vi "FC_Parse_Comp_Info.vi"(8 "Error In":errorcluster, 10 "All Competition Data":string) -> (0 "Error Out":errorcluster, 2 "Comp Data Cluster":T1)   [LabVIEW 2014, in "FC_FIRST Client.lvlib"]
doc: "This VI parses the data of a competition and returns a cluster of the competition attributes"
uses:
  FC_FIRST Client.lvlib
  FC_Competition Attributes.ctl
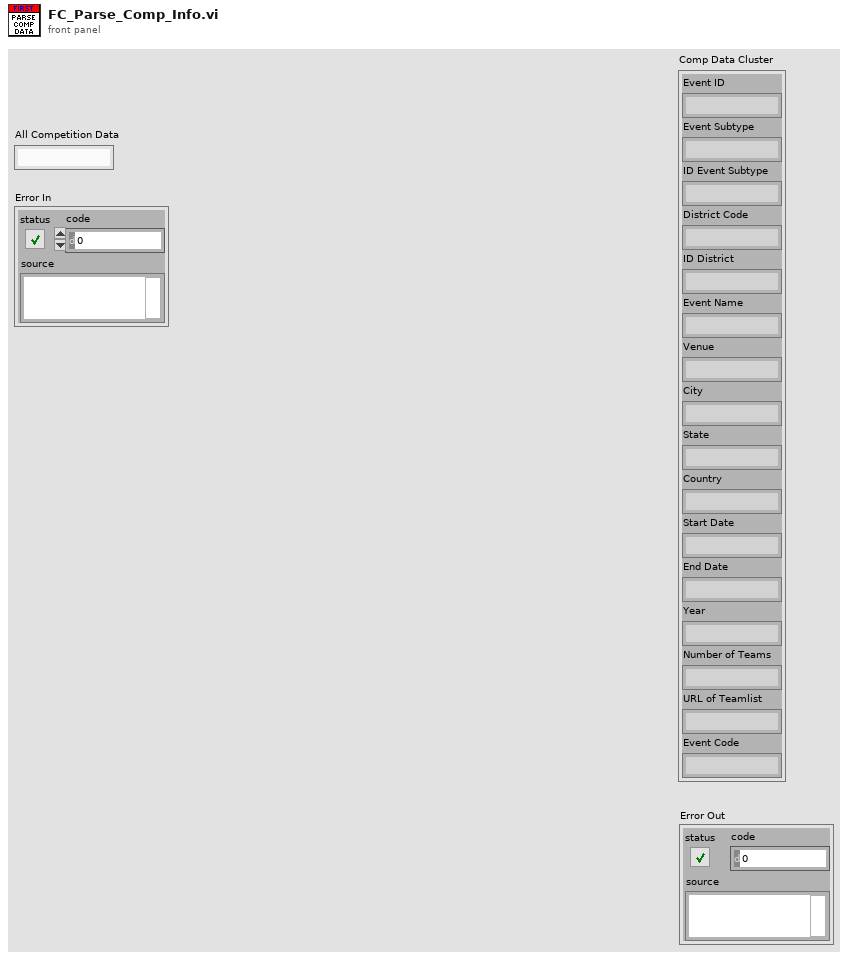
[diagram p1: front panel]
types:
  T1 = typedef "FC_FIRST Client.lvlib/FC_Competition Attributes.ctl" = cluster{"Event ID":string, "Event Subtype":string, "ID Event Subtype":string, "District Code":string, "ID District":string, "Event Name":string, "Venue":string, "City":string, "State":string, "Country":string, "Start Date":string, "End Date":string, "Year":string, "Number of Teams":string, "URL of Teamlist":string, "Event Code":string}
  T2 = cluster{"[0]":string, "[1]":string, "[2]":string, "[3]":string, "[4]":string, "[5]":string, "[6]":string, "[7]":string, "[8]":string, "[9]":string, "[10]":string, "[11]":string, "[12]":string, "[13]":string, "[14]":string, "[15]":string}
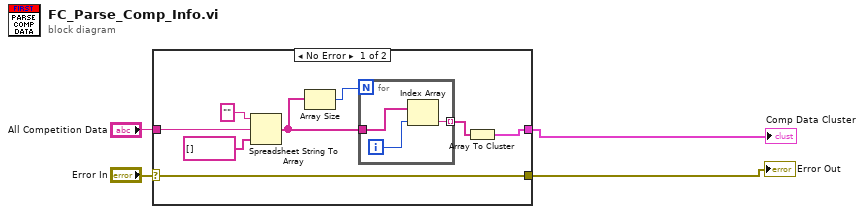
[diagram p0: block diagram]
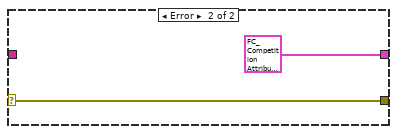
[diagram p2: hidden frame]
diagram:
  n1 = case shown="No Error" "Error In" {
    selector: "Error In" -> [w9 w17]
    tunnel: "All Competition Data" -> [w10 _]
    tunnel: [w9 w17] -> w1
    tunnel: [w5 T1 {"Event ID"="", "Event Subtype"="", "ID Event Subtype"="", "District Code"="", "ID District"="", "Event Name"="", "Venue"="", "City"="", "State"="", "Country"="", "Start Date"="", "End Date"="", "Year"="", "Number of Teams"="", "URL of Teamlist"="", "Event Code"=""} ("Comp Data Cluster")] -> w2
    frame No Error {
      n2 = Spreadsheet String To Array(format string="", spreadsheet string=w10, array type (2D Dbl)=string[] []) -> (array=w7:string[])  [unwired: 1 in]
      n3 = Array Size(array=w7) -> (size(s)=w8:i32)
      n4 = for {
        N: w8 -> [_]
        tunnel: w7 -> [w14]
        tunnel: [w13] -> w6 mode=indexing
        i -> [w15]
        n5 = Index Array(array=w14, index=w15) -> (element=w13:string)
      }
      n6 = Array To Cluster(array=w6) -> (cluster=w5:T2)
    }
    frame Error {
    }
  }
  "Error Out" <- w1
  "Comp Data Cluster" <- w2
